vi "target - single rate - variables.vi"   [LabVIEW 2012]
uses:
  <vilib>/Platform/TimedLoop/XDataNode/timing_clust.ctl
  <vilib>/Platform/TimedLoop/XDataNode/nitl_modes.ctl
  <vilib>/Platform/TimedLoop/XDataNode/wakeup.ctl
  <vilib>/Platform/TimedLoop/XDataNode/XDataNode.xnode
  <vilib>/Platform/TimedLoop/XDataNode/XDNodeRunTimeDep.lvlib
panel:
  # "The Network Variable Engine and Variable Client Support must be installed on the RT target\nfor this application to function properly. If the Network Variable Engine is not supported on\nthe target (e.g.  FP-2000 with <32MB of RAM), open the project and move the variable library\nto My Computer in the project. Doing this will deploy the variables to localhost but\nwill still require that Variable Client Support be installed on the RT target."
types:
  T1 = typedef "XDNodeRunTimeDep.lvlib/timing_clust.ctl" = cluster{"Expected End [f-1]":u64, "Actual End [f-1]":u64, "Finished Late? [f-1]":bool, "Expected End [i-1]":u64, "Actual End [i-1]":u64, "Finished Late? [i-1]":bool, "Expected Start [i]":u64, "Actual Start [i]":u64, "Expected Start [f]":u64, "Actual Start [f]":u64, "Source Name":string, "Structure Name":string, "Period":i64, "Deadline":i64, "Offset":i64, "Start":i64, "Priority":i32, "Timeout":i32, "Mode":T2, "Wakeup Reason":T3, "Error":errorcluster, "Source Type":string, "Secondary Source Type":string, "Global End Time":u64, "Global Start Time":u64, "Frame Duration":u64, "Iteration Duration":u64, "Assigned CPU":i32, "I/O Scan Engine Mode":u32}
  T2 = typedef "XDNodeRunTimeDep.lvlib/nitl_modes.ctl" = enum32{"No Change", "Process missed periods, maintain original phase", "Discard missed periods, maintain original phase", "Process missed periods, ignore original phase", "Discard missed periods, ignore original phase"}
  T3 = typedef "XDNodeRunTimeDep.lvlib/wakeup.ctl" = enum32{"Normal", "Aborted", "Asynchronous wakeup", "Timing source error", "Timed loop error", "Timeout"}
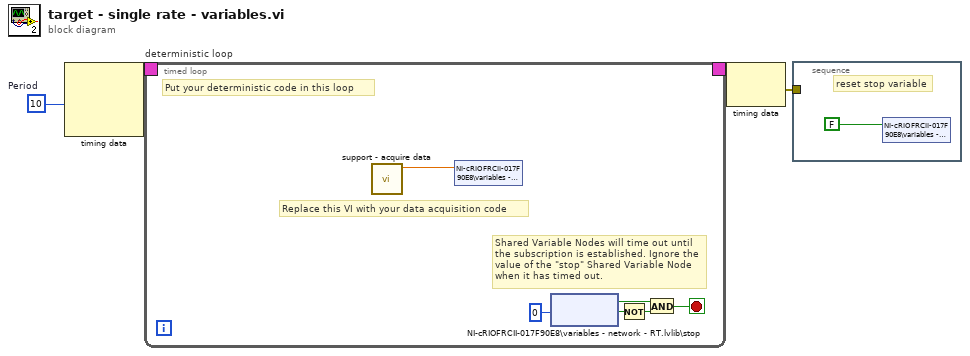
[diagram p0: block diagram]
diagram:
  w2 = i64 10  # Period
  n1 = node-c288 ("Input Node")(w2) -> (w4:T1)  [unwired: 2 in]
  n2 = timed-loop "deterministic loop" {
    timing: w4 -> [_]
    timing-out: [_] -> w3
    stop <- w9 stop-if-true
    # "Shared Variable Nodes will time out until the subscription is established. Ignore the value of the \"stop\" Shared Variable Node when it has timed out."
    # "Replace this VI with your data acquisition code"
    # "Put your deterministic code in this loop"
    n3 = call <resource>:"support - acquire data.vi"() -> ("sin(x)"=w10:dbl)  [unwired: 10 in, 1 out]
    n4 = shared-variable "NI-cRIOFRCII-017F90E8\\variables - network - RT.lvlib\\data"(w10) -> ()  [unwired: 1 in, 1 out]
    n5 = shared-variable "NI-cRIOFRCII-017F90E8\\variables - network - RT.lvlib\\stop"(0 ("ms timeout (0)")) -> (w6:bool, w7:bool)  [unwired: 1 in, 1 out]
    n6 = Not(x=w7) -> (.not. x?=w8:bool)
    n7 = And(x=w6, y=w8) -> (x .and. y?=w9:bool)
  }
  n8 = node-c288 ("Output Node")(w3) -> (w1:errorcluster)
  n9 = stacked-sequence {
    tunnel: w1 -> [_]
    frame #0 {
      # "reset stop variable"
      n10 = shared-variable "NI-cRIOFRCII-017F90E8\\variables - network - RT.lvlib\\stop"(FALSE) -> ()  [unwired: 1 in, 1 out]
    }
  }
